vi "Read Calibration 1.vi"(8 "error in (no error)":errorcluster, 11 "RP Instrument in":refnum<class "RP Instrument.lvclass">) -> (0 "error out":errorcluster, 2 "RP EEPROM Calibration":T1 {"magic" format="%x"}, 3 "RP Instrument out":refnum<class "RP Instrument.lvclass">)   [LabVIEW 2018, in "RP Instrument.lvclass"]
uses:
  RP Instrument.lvclass
  RP EEPROM Calibration.ctl
  RP Instrument.lvclass/RP Instrument.ctl
  RP Communicator/RP Communicator.lvclass/RP Communicator.ctl
  RP Communicator/Read RP EEPROM Calibration.vi
  RP Communicator/RP Communicator.lvclass
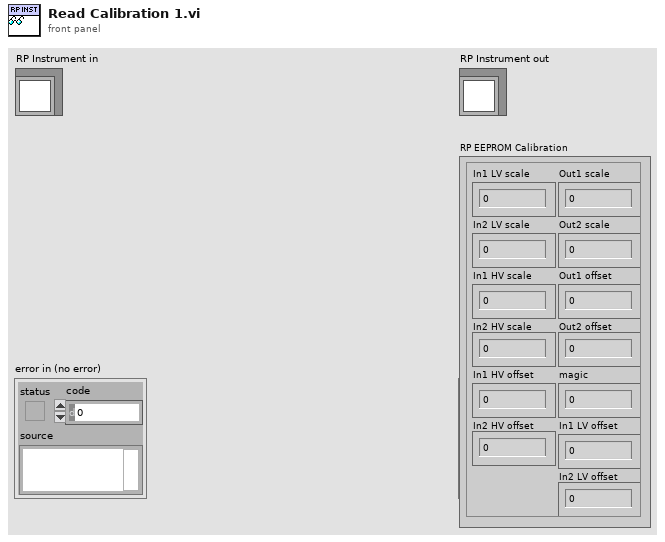
[diagram p1: front panel]
types:
  T1 = typedef "RP EEPROM Calibration.ctl" = cluster{"In1 LV scale":u32, "In2 LV scale":u32, "In1 HV scale":u32, "In2 HV scale":u32, "In1 HV offset":i32, "In2 HV offset":i32, "Out1 scale":u32, "Out2 scale":u32, "Out1 offset":i32, "Out2 offset":i32, "magic":u32, "In1 LV offset":i32, "In2 LV offset":i32}
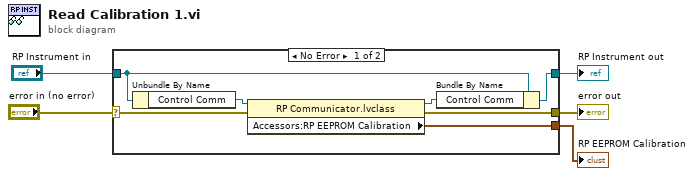
[diagram p0: block diagram]
diagram:
  n1 = case shown="No Error" "error in (no error)" {
    selector: "error in (no error)" -> [w7 w13]
    tunnel: [w6 w13] -> w4
    tunnel: [w9 w14] -> w2
    tunnel: "RP Instrument in" -> [w12 w14]
    tunnel: [w10 _] -> w1
    frame No Error {
      n2 = Unbundle By Name(w12) -> ("Control Comm"=w11:refnum<class "RP Communicator.lvclass">)
      n3 = property class="RP Communicator.lvclass"(reference=w11, error in=w7) -> (reference out=w8:refnum<class "RP Communicator.lvclass">, error out=w6:errorcluster, "Accessors:RP EEPROM Calibration"=w10:T1)
      n4 = Bundle By Name(cluster=w12, "Control Comm"=w8) -> (w9:refnum<class "RP Instrument.lvclass">)
    }
    frame Error {
    }
  }
  "error out" <- w4
  "RP Instrument out" <- w2
  "RP EEPROM Calibration" <- w1
